vi "Final Msgs.vi"(10 "Event Ref":refnum<event-registration>) -> (2 "Final Msgs":refnum<class "Msg.lvclass">[](array[class]))   [LabVIEW 2020, in "jettl.lvlib" / "Actor.lvlib"]
uses:
  Actor.lvlib
  Msg/Msg.lvclass
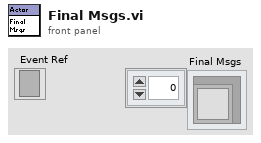
[diagram p1: front panel]
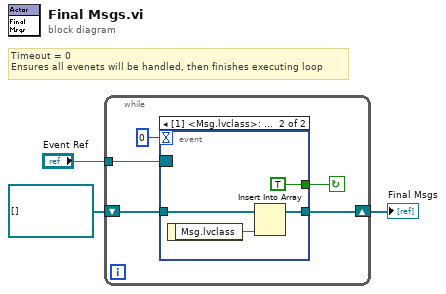
[diagram p0: block diagram]
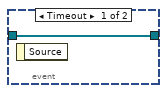
[diagram p2: hidden frame]
diagram:
  # "Timeout = 0\nEnsures all evenets will be handled, then finishes executing loop"
  n1 = while {
    shift-right: [w7] -> w1
    shift-left: refnum<class "Msg.lvclass">[] [] -> [w8]
    tunnel: "Event Ref" -> [w6]
    stop <- w5 continue-if-true
    n2 = event shown="[1] <Msg.lvclass>: User Event" {
      selector: w6 -> [_ _]
      dyn-events: _ -> [_ _]
      timeout: 0 -> [_ _]
      tunnel: w8 -> [w9 w13]
      tunnel: [w9 w12] -> w7
      tunnel: [_ TRUE] -> w5
      event Timeout {
        n3 = event-data() -> ()  [unwired: 1 in, 1 out]
      }
      event User Event {
        n4 = event-data() -> ("Msg.lvclass"=w11:refnum<class "Msg.lvclass">)  [unwired: 1 in]
        n5 = Insert Into Array(array=w13, new element=w11) -> (w12:refnum<class "Msg.lvclass">[])  [unwired: 1 in]
      }
    }
  }
  "Final Msgs" <- w1
